vi "NXT_DisplayLine.vi"(7 "Clear Display (F)":bool, 9 "End Location":cluster{"X":i16, "Y":i16}, 10 "Start Location":cluster{"X":i16, "Y":i16}, 11 "Sequence Flow in":T2) -> (3 "Sequence Flow out":T2)   [LabVIEW 2009]
doc: "Draws a line on the NXT display."
uses:
  Library.llb/SequenceBoolean.ctl
  Library.llb/NXTSyscallRefnum.ctl
  C:/Program Files/National Instruments/LabVIEW 2009/resource/objmgr/NXTInputOutput.rc
panel:
  in  "Generic Refnum Name":T1
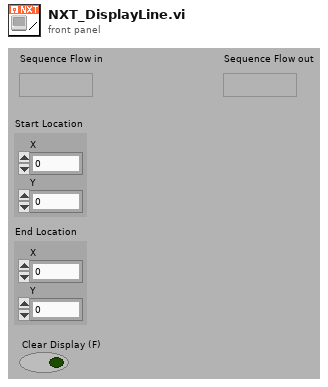
[diagram p1: front panel]
types:
  T1 = typedef "NXTSyscallRefnum.ctl" = refnum<k21>
  T2 = typedef "SequenceBoolean.ctl" = bool
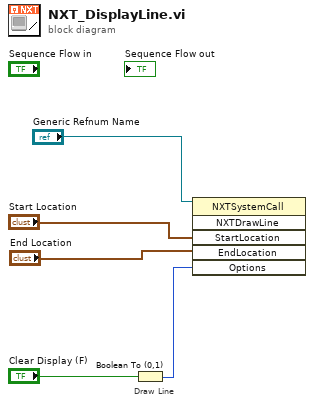
[diagram p0: block diagram]
diagram:
  # "Draw Line"
  n1 = Boolean To (0,1)(Boolean="Clear Display (F)") -> (0, 1=w2:i16)
  n2 = invoke class="NXTSystemCall" method="NXTDrawLine"(reference="Generic Refnum Name", "StartLocation"="Start Location", "EndLocation"="End Location", "Options"=w2) -> ()  [unwired: 2 in, 6 out]
